vi "Temperature Grad Read Array.vi"(8 "error in":errorcluster, 11 "Chiller in":refnum<class "Chiller.lvclass">) -> (0 "error out":errorcluster, 1 "Changed or First Call?":bool, 2 "Temperature SP":dbl[](array[numeric]), 3 "Chiller out":refnum<class "Chiller.lvclass">)   [LabVIEW 2023, in "Chiller.lvclass"]
uses:
  Chiller.lvclass
  Low Level Capabilities/Temperature/Temperature Gradient/Temperature Gradient.lvclass
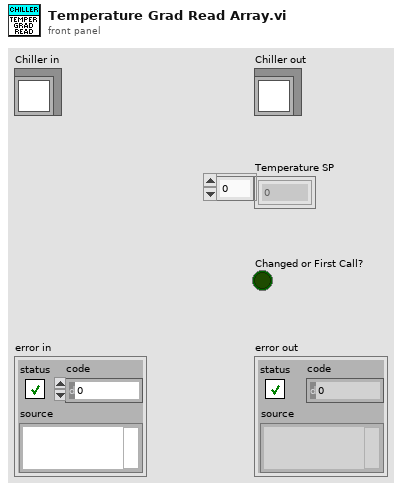
[diagram p1: front panel]
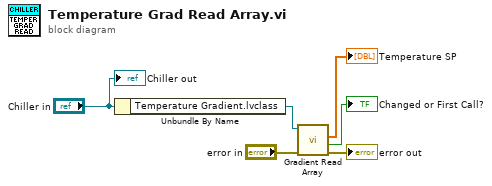
[diagram p0: block diagram]
diagram:
  n1 = Unbundle By Name("Chiller in") -> ("Temperature Gradient.lvclass"=w6:refnum<class "Temperature Gradient.lvclass">)
  n2 = call-dynamic "Gradient Read Array.vi"("error in"="error in", "Temperature Gradient in"=w6) -> ("error out"=→"error out":errorcluster, "Changed or First Call?"=→"Changed or First Call?":bool, "Temperature SP"=→"Temperature SP":dbl[])  [unwired: 6 in, 1 out]
  "Chiller out" <- "Chiller in"
